vi "Matrix-Vector_mult_loop.vi"(7 "Row":refnum<k21>="AasCol", 9 "Ns":u16=9, 11 "X":sgl[](array[numeric])=[0.0, 0.0, 0.0, 0.0, 0.0, 0.0, 0.0, 0.0, 0.0, 0.0, 0.0, 0.0, 0.0, 0.0, 0.0, 0.0, 0.0, 0.0, 0.0, 0.0, 0.0, 0.0, 0.0, 0.0, 0.0]) -> (2 "A x X":sgl[](array[numeric]))   [LabVIEW 2017]
doc: "Multiplies <B>Matrix A</B> by an input <B>Vector b</B>. This operation is useful for FPGA control applications, such as state-feedback control. You can use more than one multiplier to reduce the latency of this operation. To define <B>Matrix A</B>, double-click this Express VI and use the <B>Matrix Data Initialization</B> page to specify a VI, TXT, or CSV file that contains the matrix data. If you do not define <B>Matrix A</B>, this Express VI uses a matrix of zeroes instead.\n--------------------\n\nThis Express VI is configured as follows:\n\n<b>Fixed-Point Configuration</b>\nMatrix A Type: <+/-,32,16>\nVector b Type: <+/-,32,16>\nVector c Type: <+/-,64,36>\nOverflow mode: Truncate [Not Needed]\nRounding mode: Saturate [Not Needed]\n\n<b>Matrix A Configuration</b>\nMatrix Dimensions: 9 * 9\n\n<b>Multiplier Configuration</b>\nNumber of multipliers: 9\nNumber of multiplier pipeline stages: 0\n\n<b>Implementation</b>\nMatrix Vector Multiplication: 11 cycles"
uses:
  <vilib>/fxp/LVFixedPointOverflowPolicyTypeDef.ctl
  <vilib>/fxp/LVFixedPointQuantizationPolicyTypeDef.ctl
  <vilib>/rvi/Analysis/control/MatrixVector/Matrix Vector subs/niFPGAMatrixVector_TargetState.ctl
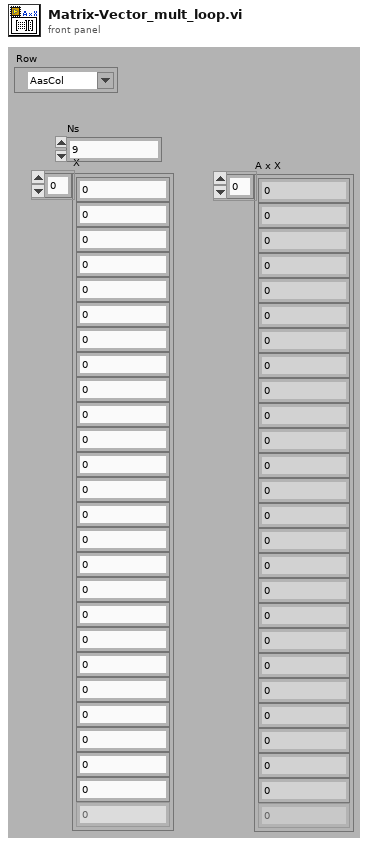
[diagram p1: front panel]
types:
  T1 = typedef "niFPGAMatrixVector_TargetState.ctl" = cluster{"matrix datatype":cluster{"sign?":bool, "word length":i32, "integer word length":i32}, "vector datatype":cluster{"sign?":bool, "word length":i32, "integer word length":i32}, "result datatype":cluster{"sign?":bool, "word length":i32, "integer word length":i32}, "matrix size":cluster{"matrix rows":i32, "matrix columns":i32}, "Adapt to source":bool, "Matrix A constant?":bool, "# multipliers":i32, "# number of multiplier pipeline":i32, "Overflow mode":T2, "Rounding mode":T3, "Initialization method":u16, "File path conversion":path, "Matrix data":ext[][], "Code generated":bool}
  T2 = typedef "LVFixedPointOverflowPolicyTypeDef.ctl" = enum32{"Wrap", "Saturate"}
  T3 = typedef "LVFixedPointQuantizationPolicyTypeDef.ctl" = enum32{"Truncate", "Round-Half-Up (Asymmetric)", "Round-Half-Even"}
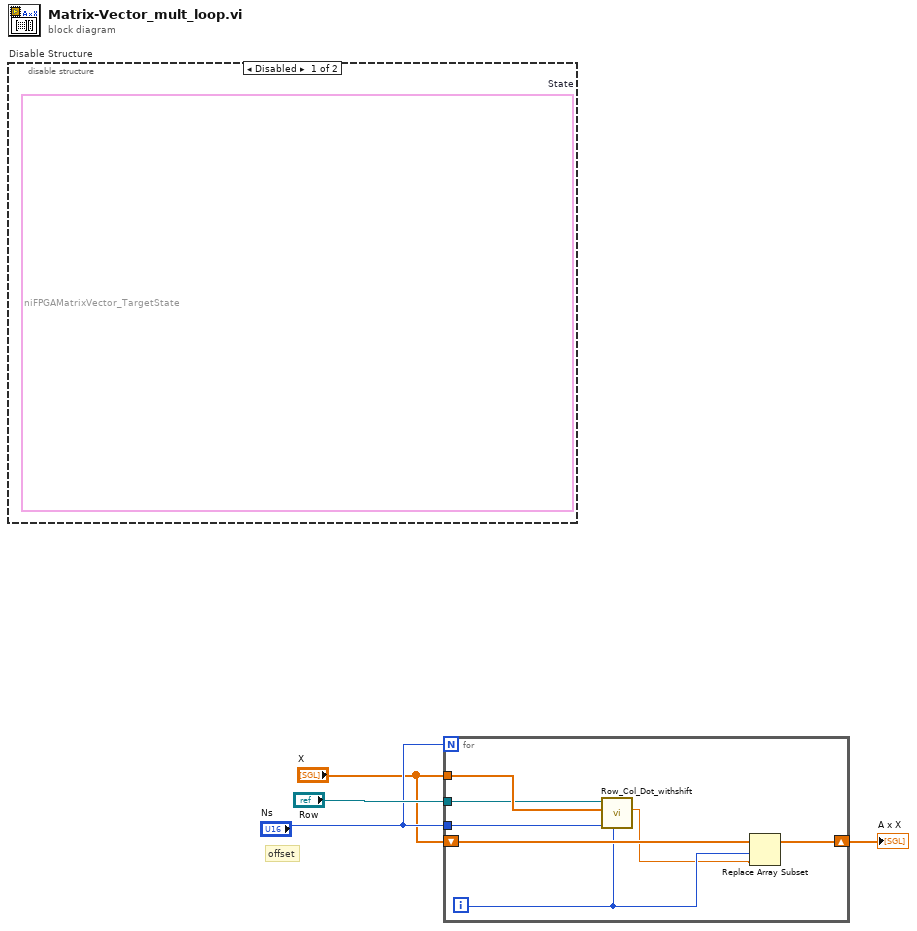
[diagram p0: block diagram]
diagram:
  # "offset"
  n1 = disable-structure "Disable Structure" shown="Disabled" {
    frame Disabled {
      (unwired) T1 {"matrix datatype"={"sign?"=TRUE, "word length"=32, "integer word length"=16}, "vector datatype"={"sign?"=TRUE, "word length"=32, "integer word length"=16}, "result datatype"={"sign?"=TRUE, "word length"=64, "integer word length"=36}, "matrix size"={"matrix rows"=9, "matrix columns"=9}, "Adapt to source"=TRUE, "Matrix A constant?"=TRUE, "# multipliers"=9, "# number of multiplier pipeline"=0, "Overflow mode"=enum."Saturate", "Rounding mode"=enum."Truncate", "Initialization method"=0, "File path conversion"=path "C:/Power Electronics Design Guide/IP Cores/IP Cores - LabVIEW FPGA/HIL Solver/Initialize A Matrix.vi", "Matrix data"=[[0.0, 0.0, 0.0, 833.5, 0.0, 0.0, -833.5, 0.0, 0.0], [0.0, 0.0, 0.0, 0.0, 833.5, 0.0, 0.0, -833.5, 0.0], [0.0, 0.0, 0.0, 0.0, 0.0, 833.5, 0.0, 0.0, -833.5], [-1250.0, 0.0, 0.0, 0.0, 0.0, 0.0, 0.0, 0.0, 0.0], [0.0, -1250.0, 0.0, 0.0, 0.0, 0.0, 0.0, 0.0, 0.0], [0.0, 0.0, -1250.0, 0.0, 0.0, 0.0, 0.0, 0.0, 0.0], [500.0, 0.0, 0.0, 0.0, 0.0, 0.0, -2500.0, 0.0, 0.0], [0.0, 500.0, 0.0, 0.0, 0.0, 0.0, 0.0, -2500.0, 0.0], [0.0, 0.0, 500.0, 0.0, 0.0, 0.0, 0.0, 0.0, -2500.0]], "Code generated"=TRUE}  # State
    }
    frame Enabled {
    }
  }
  n2 = for {
    N: "Ns" -> [_]
    tunnel: "Row" -> [w9]
    tunnel: "X" -> [w10]
    tunnel: "Ns" -> [w11]
    shift-right: [w8] -> w2
    shift-left: "X" -> [w7]
    i -> [w6]
    n3 = call "Row_Col_Dot_withshift.vi"("Shift"=w6, "NS"=w11, "X"=w10, "Refnum in"=w9) -> ("a^t*x"=w5:sgl)  [unwired: 7 in]
    n4 = Replace Array Subset(array=w7, new element=w5, index=w6) -> (w8:sgl[])
  }
  "A x X" <- w2
